vi "loop_on_pic.vi"(10 "Y Resolution":i32=600, 11 "X Resolution":i32=800) -> (0 "error out":errorcluster, 3 "Image Pixels (U8)":u8[][][](array[numeric]))   [LabVIEW 2025]
uses:
  <vilib>/vision/NI_Vision_Development_Module.lvlib
panel:
  out "Image":T1(plugin-control)
  out "Image Pixels (Float)":sgl[][][](array[numeric])
  out "appended path":path
  out "filenames":string[](array[string])
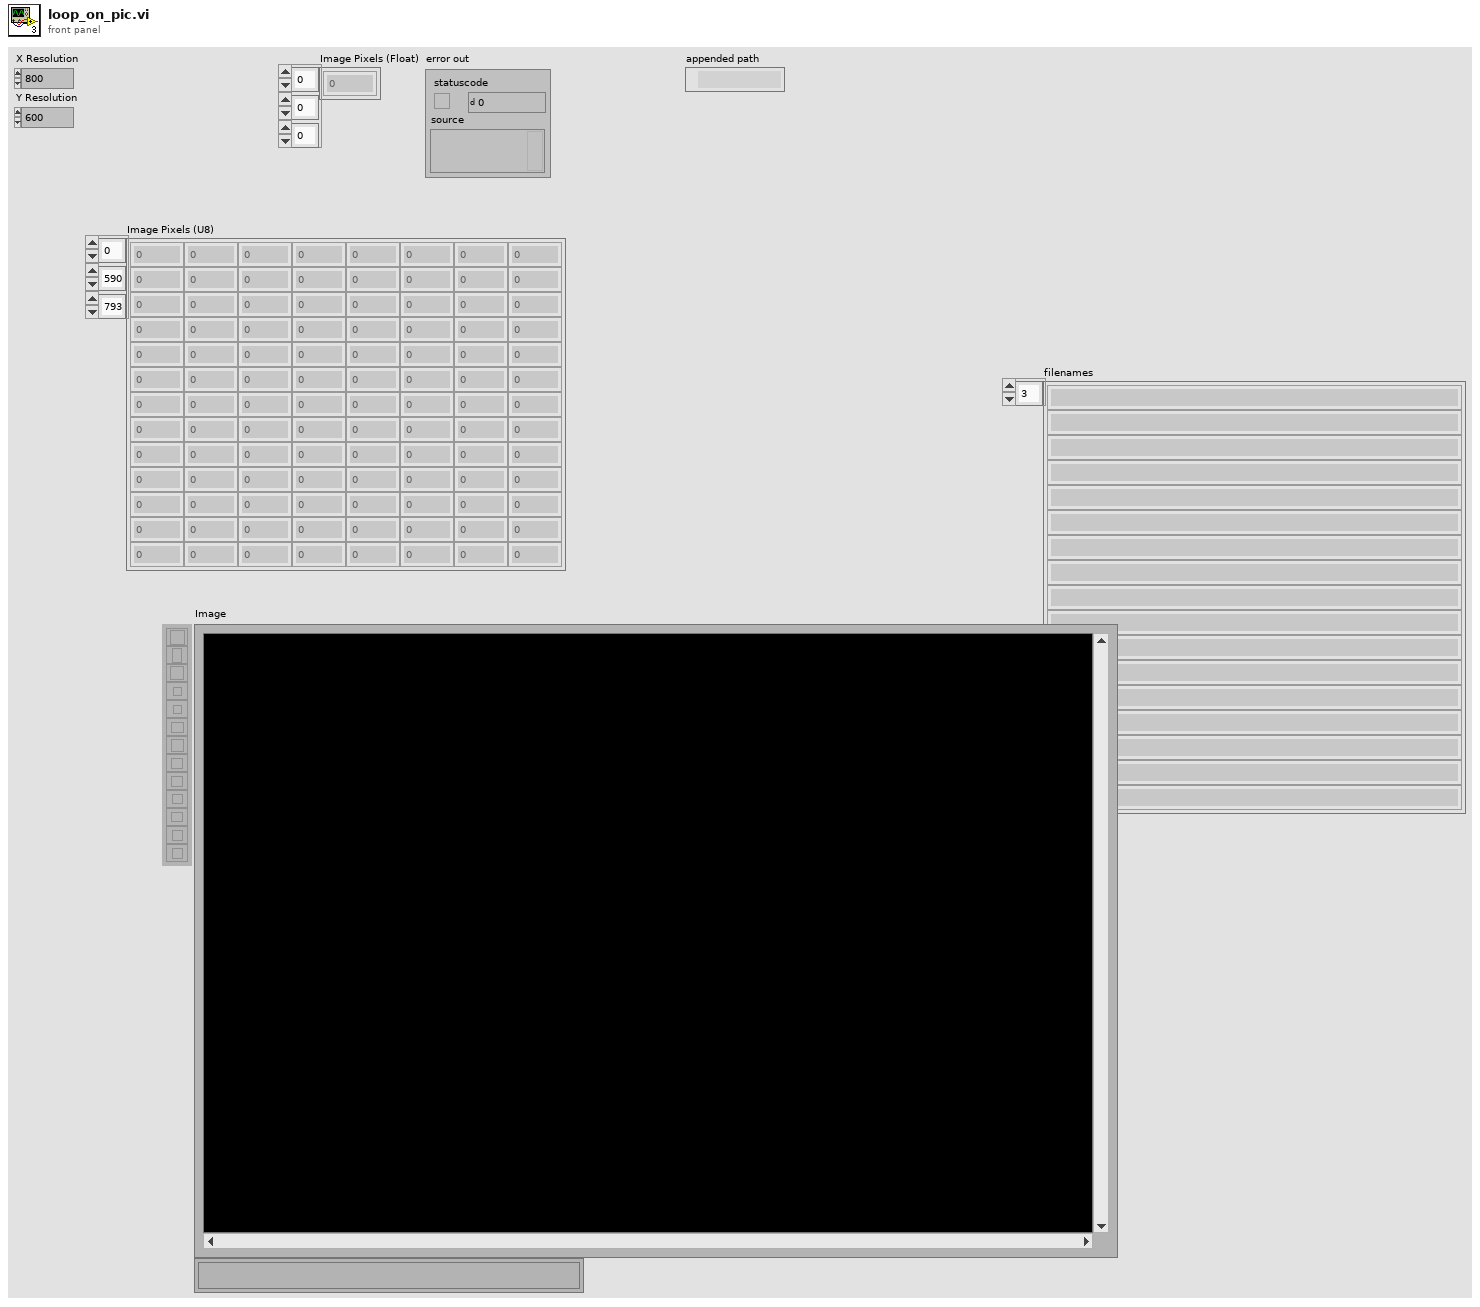
[diagram p1: front panel]
types:
  T1 = typedef "IMAQ Image.ctl" = refnum<image>
  T2 = typedef "Image Type" = u32
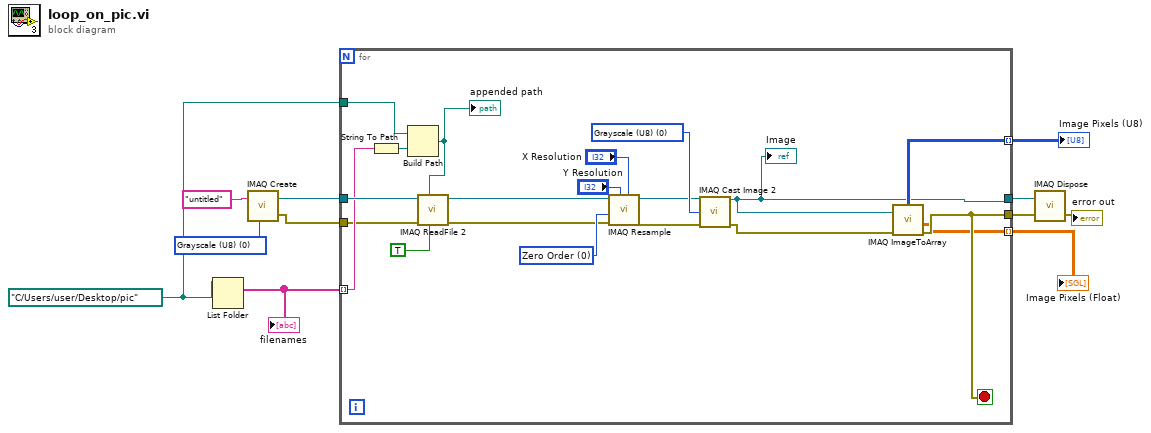
[diagram p0: block diagram]
diagram:
  w9 = T2 0 items=["Grayscale (U8)", "Grayscale (I16)", "Grayscale (SGL)", "Complex (CSG)", "RGB (U32)", "HSL (U32)", "RGB (U64)", "Grayscale (U16)"] ("Image Type")
  w10 = path "C:/Users/user/Desktop/pic" ("path")
  n1 = List Folder(path=w10) -> (filenames=w4:string[])  [unwired: 3 in, 3 out]
  "filenames" <- w4
  n2 = call "IMAQ Create"("Image Name"="untitled", "Image Type"=w9) -> ("New Image"=w11:T1, "error out"=w7:errorcluster)  [unwired: 3 in]
  n3 = for {
    tunnel: w11 -> [w31]
    tunnel: w4 -> [w28] mode=indexing
    tunnel: w10 -> [w29]
    tunnel: w7 -> [w26]
    tunnel: [w12] -> w6
    tunnel: [w25] -> w5
    tunnel: [w23] -> w2 mode=indexing
    tunnel: [w20] -> w1 mode=indexing
    stop <- w25 stop-if-true
    w16 = u32 0 items=["Zero Order", "Bi-Linear", "Quadratic", "Cubic Spline"] ("Interpolation Type")
    w21 = T2 0 items=["Grayscale (U8)", "Grayscale (I16)", "Grayscale (SGL)", "Complex (CSG)", "RGB (U32)", "HSL (U32)", "RGB (U64)", "Grayscale (U16)"] ("Image Type")
    n4 = String To Path(string=w28) -> (path=w27:path)
    n5 = Build Path(base path=w29, name or relative path=w27) -> (appended path=w24:path)
    "appended path" <- w24
    n6 = call "IMAQ ReadFile 2"("Use File Path Image Type"=TRUE, "File Path"=w24, "error in (no error)"=w26, "Image"=w31) -> ("error out"=w15:errorcluster, "Image Out"=w19:T1)  [unwired: 3 in, 3 out]
    n7 = call "IMAQ Resample"("X Resolution"="X Resolution", "Y Resolution"="Y Resolution", "error in (no error)"=w15, "Interpolation Type"=w16, "Image Src"=w19) -> ("error out"=w17:errorcluster, "Image Dst Out"=w18:T1)  [unwired: 5 in]
    n8 = call "IMAQ Cast Image 2"("Image Src"=w18, "Image Type"=w21, "error in (no error)"=w17) -> ("Image Dst Out"=w12:T1, "error out"=w22:errorcluster)  [unwired: 11 in]
    "Image" <- w12
    n9 = call "IMAQ ImageToArray"("error in (no error)"=w22, "Image"=w12) -> ("Image Pixels (Float)"=w23:sgl[][], "error out"=w25:errorcluster, "Image Pixels (U8)"=w20:u8[][])  [unwired: 2 in, 2 out]
  }
  "Image Pixels (U8)" <- w1
  "Image Pixels (Float)" <- w2
  n10 = call "IMAQ Dispose"("Image"=w6, "error in (no error)"=w5) -> ("error out"=→"error out":errorcluster)  [unwired: 4 in]
